vi "3_Navigation and Editing(170382)(170307).vi"() -> ()   [LabVIEW 2015]
doc: "This VI is an exercise for you to practice editing front panel objects. You can follow the different steps to this exercise by reading along in your LabVIEW Tutorial Chapter 1."
panel:
  in  "Gauge":dbl(knob) scale=0.0..50.0
  in  "?":bool
  in  "?":bool
  in  "?":bool
  in  "?":bool
  out "I'm a Round LED\nResize me":bool
  out "?":dbl format="%.2f"
  in  "?":bool
  in  "?":bool
  in  "?":bool
  in  "?":bool
  in  "Digital control (owned label)\nReposition me.":dbl format="%.2f"
  # "my lABEL"
  # "Reposition the 4 slide switches above\nas a group."
  # "I'm a Free label\nDuplicate me"
  # "I'm a Free label\nDuplicate me"
  # "I'm also a Free label\nChange my font size"
  # "Place the 4 button switches above so they are\nlined up horizontally and evenly spaced apart."
  # "Resize, change the range, and\ndisplay the selected value"
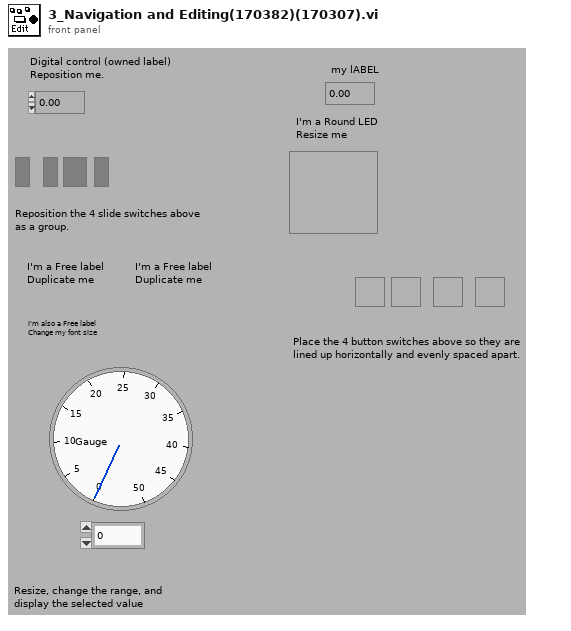
[diagram p1: front panel]
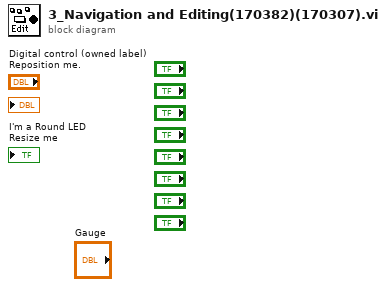
[diagram p0: block diagram]
diagram:
